vi "TP_OP_Queue.vi"(6 "max queue size (-1, unlimited)":i32=-1, 7 "OP_Queue (get queue)":T2(ring)=enum."Get Queue", 8 "error in":errorcluster) -> (0 "error out":errorcluster, 3 "Queues":T1)   [LabVIEW 2012]
doc: "Queue Management"
uses:
  controls/TP_Queues.ctl
  controls/TP_Message data.ctl
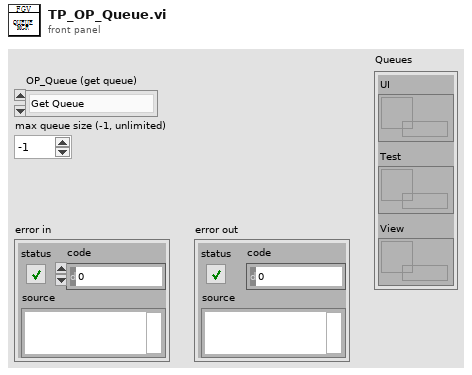
[diagram p1: front panel]
types:
  T1 = typedef "TP_Queues.ctl" = cluster{"UI":refnum<queue>, "Test":refnum<queue>, "View":refnum<queue>}
  T2 = enum16{"Create Queue", "Get Queue", "Destory Queue"}
  T3 = typedef "TP_Message data.ctl" = cluster{"CMD":string, "Paras":variant}
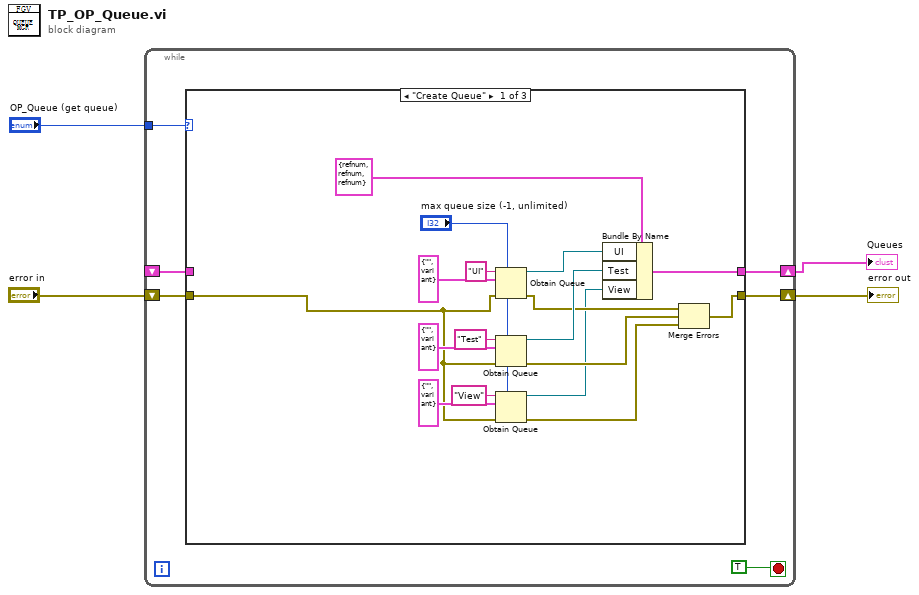
[diagram p0: block diagram]
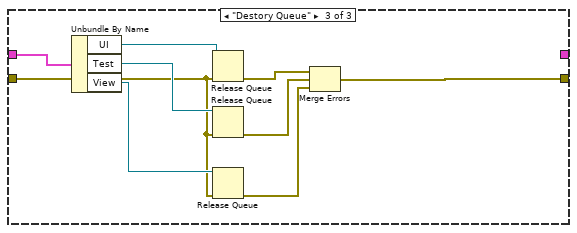
[diagram p3: hidden frame]
diagram:
  n1 = while {
    tunnel: "OP_Queue (get queue)" -> [w9]
    shift-right: [w7] -> w3
    shift-left: "error in" -> [w8]
    shift-right: [w6] -> w1
    shift-left: _ -> [w5]
    stop <- TRUE stop-if-true
    n2 = case shown="\"Create Queue\"" w9 {
      tunnel: [w21 w28 _] -> w6
      tunnel: w8 -> [w15 w29 w31]
      tunnel: [w18 w29 w33] -> w7
      tunnel: w5 -> [_ w28 w38]
      frame "Create Queue" {
        n3 = Obtain Queue(max queue size (-1, unlimited)="max queue size (-1, unlimited)", name (unnamed)="UI", element data type=T3 {"CMD"="", "Paras"=variant} ("Message"), error in (no error)=w15) -> (queue out=w23:refnum<queue>, error out=w20:errorcluster)  [unwired: 1 in, 1 out]
        n4 = Obtain Queue(max queue size (-1, unlimited)="max queue size (-1, unlimited)", name (unnamed)="Test", element data type=T3 {"CMD"="", "Paras"=variant} ("Message"), error in (no error)=w15) -> (queue out=w22:refnum<queue>, error out=w19:errorcluster)  [unwired: 1 in, 1 out]
        n5 = Obtain Queue(max queue size (-1, unlimited)="max queue size (-1, unlimited)", name (unnamed)="View", element data type=T3 {"CMD"="", "Paras"=variant} ("Message"), error in (no error)=w15) -> (queue out=w12:refnum<queue>, error out=w13:errorcluster)  [unwired: 1 in, 1 out]
        n6 = Bundle By Name(cluster=T1 {"UI"=refnum, "Test"=refnum, "View"=refnum} ("Queues"), "UI"=w23, "Test"=w22, "View"=w12) -> (w21:T1)
        n7 = Merge Errors(w20, w19, w13) -> (w18:errorcluster)
      }
      frame "Get Queue", Default {
      }
      frame "Destory Queue" {
        n8 = Unbundle By Name(w38) -> ("UI"=w37:refnum<queue>, "Test"=w36:refnum<queue>, "View"=w32:refnum<queue>)
        n9 = Release Queue(queue=w37, error in (no error)=w31) -> (error out=w35:errorcluster)  [unwired: 1 in, 2 out]
        n10 = Release Queue(queue=w36, error in (no error)=w31) -> (error out=w34:errorcluster)  [unwired: 1 in, 2 out]
        n11 = Release Queue(queue=w32, error in (no error)=w31) -> (error out=w30:errorcluster)  [unwired: 1 in, 2 out]
        n12 = Merge Errors(w35, w34, w30) -> (w33:errorcluster)
      }
    }
  }
  "error out" <- w3
  "Queues" <- w1
